vi "Laser Control.vi"(0 "control_laser_source_channel_0_reference":u64 caption="Device In", 1 "control_laser_source_LED_reference":u64 caption="Device In", 2 "control_request":string, 5 "control_laser_source_channel_1_reference":u64 caption="Device In", 7 "control_laser_source_channel_2_reference":u64 caption="Device In", 9 "control_laser_source_channel_3_reference":u64 caption="Device In", 11 "control_laser_source_vibrator_reference":u64 caption="Device In", 12 "control_laser_source":string, 13 "control_laser_source_power":dbl caption="Device In") -> (3 "indicator_light_source_LED_reference":u64 caption="Phidget ID", 4 "indicator_light_source_channel_0_reference":u64 caption="Phidget ID", 6 "indicator_light_source_channel_1_reference":u64 caption="Phidget ID", 8 "indicator_light_source_channel_2_reference":u64 caption="Phidget ID", 10 "indicator_light_source_channel_3_reference":u64 caption="Phidget ID", 14 "indicator_light_source_status":bool caption="Attached?", 15 "indicator_light_source_vibrator_reference":u64 caption="Phidget ID")   [LabVIEW 2020]
uses:
  <vilib>/Utility/file.llb/Read Delimited Spreadsheet (string).vi
  <instrlib>/Phidgets/Phidget Voltage Output/Public/VoltageOutputOpen.vi
  <instrlib>/Phidgets/Phidget Digital Output/Public/DigitalOutputOpen.vi
  <instrlib>/Phidgets/Phidget Voltage Output/Public/VoltageOutputClose.vi
  <instrlib>/Phidgets/Phidget Voltage Output/Phidget Voltage Output.lvlib
  <instrlib>/Phidgets/Phidget Digital Output/Phidget Digital Output.lvlib
panel:
  out "Attached?":bool
  out "error out 12":errorcluster caption="error out"
  out "error out 11":errorcluster caption="error out"
  out "error out 10":errorcluster caption="error out"
  out "error out 9":errorcluster caption="error out"
  out "error out 8":errorcluster caption="error out"
  out "error out 7":errorcluster caption="error out"
  out "error out 6":errorcluster caption="error out"
  out "error out 5":errorcluster caption="error out"
  out "error out 4":errorcluster caption="error out"
  out "error out 3":errorcluster caption="error out"
  out "error out 2":errorcluster caption="error out"
  out "error out":errorcluster
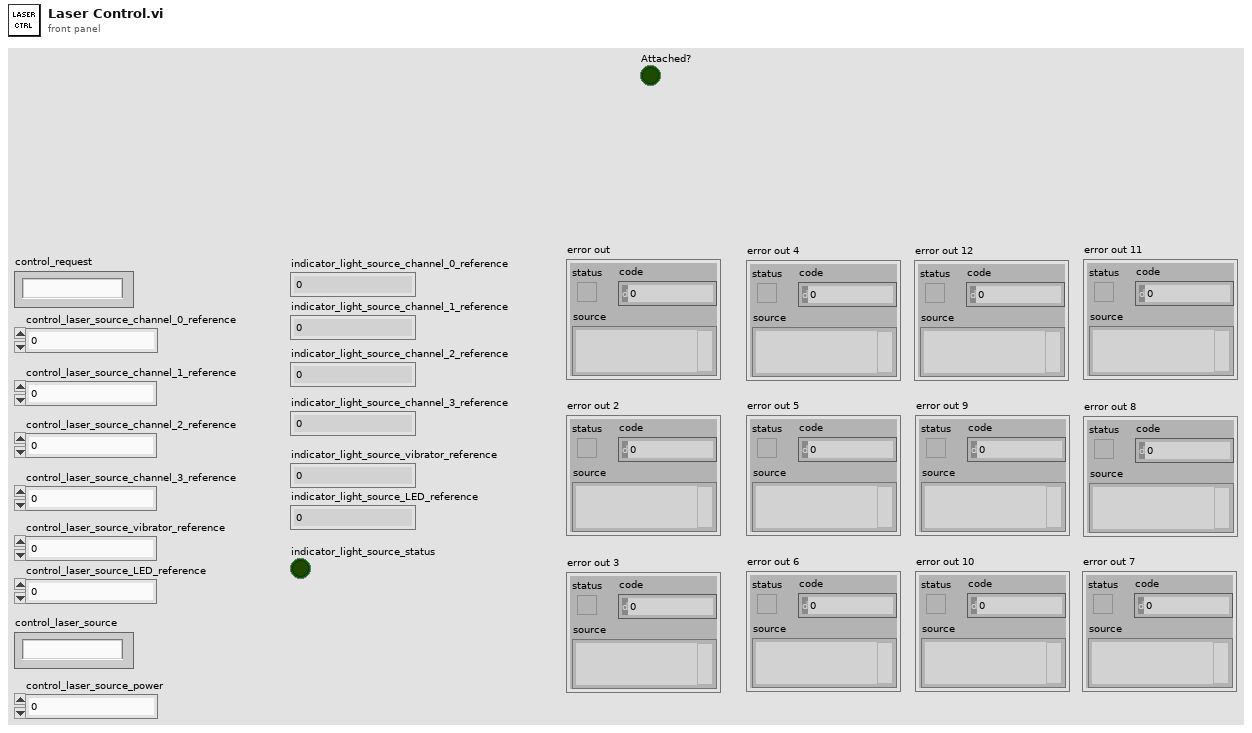
[diagram p1: front panel]
types:
  T1 = cluster{"Serial Number":i32, "Channel":i32, "Port":i32}
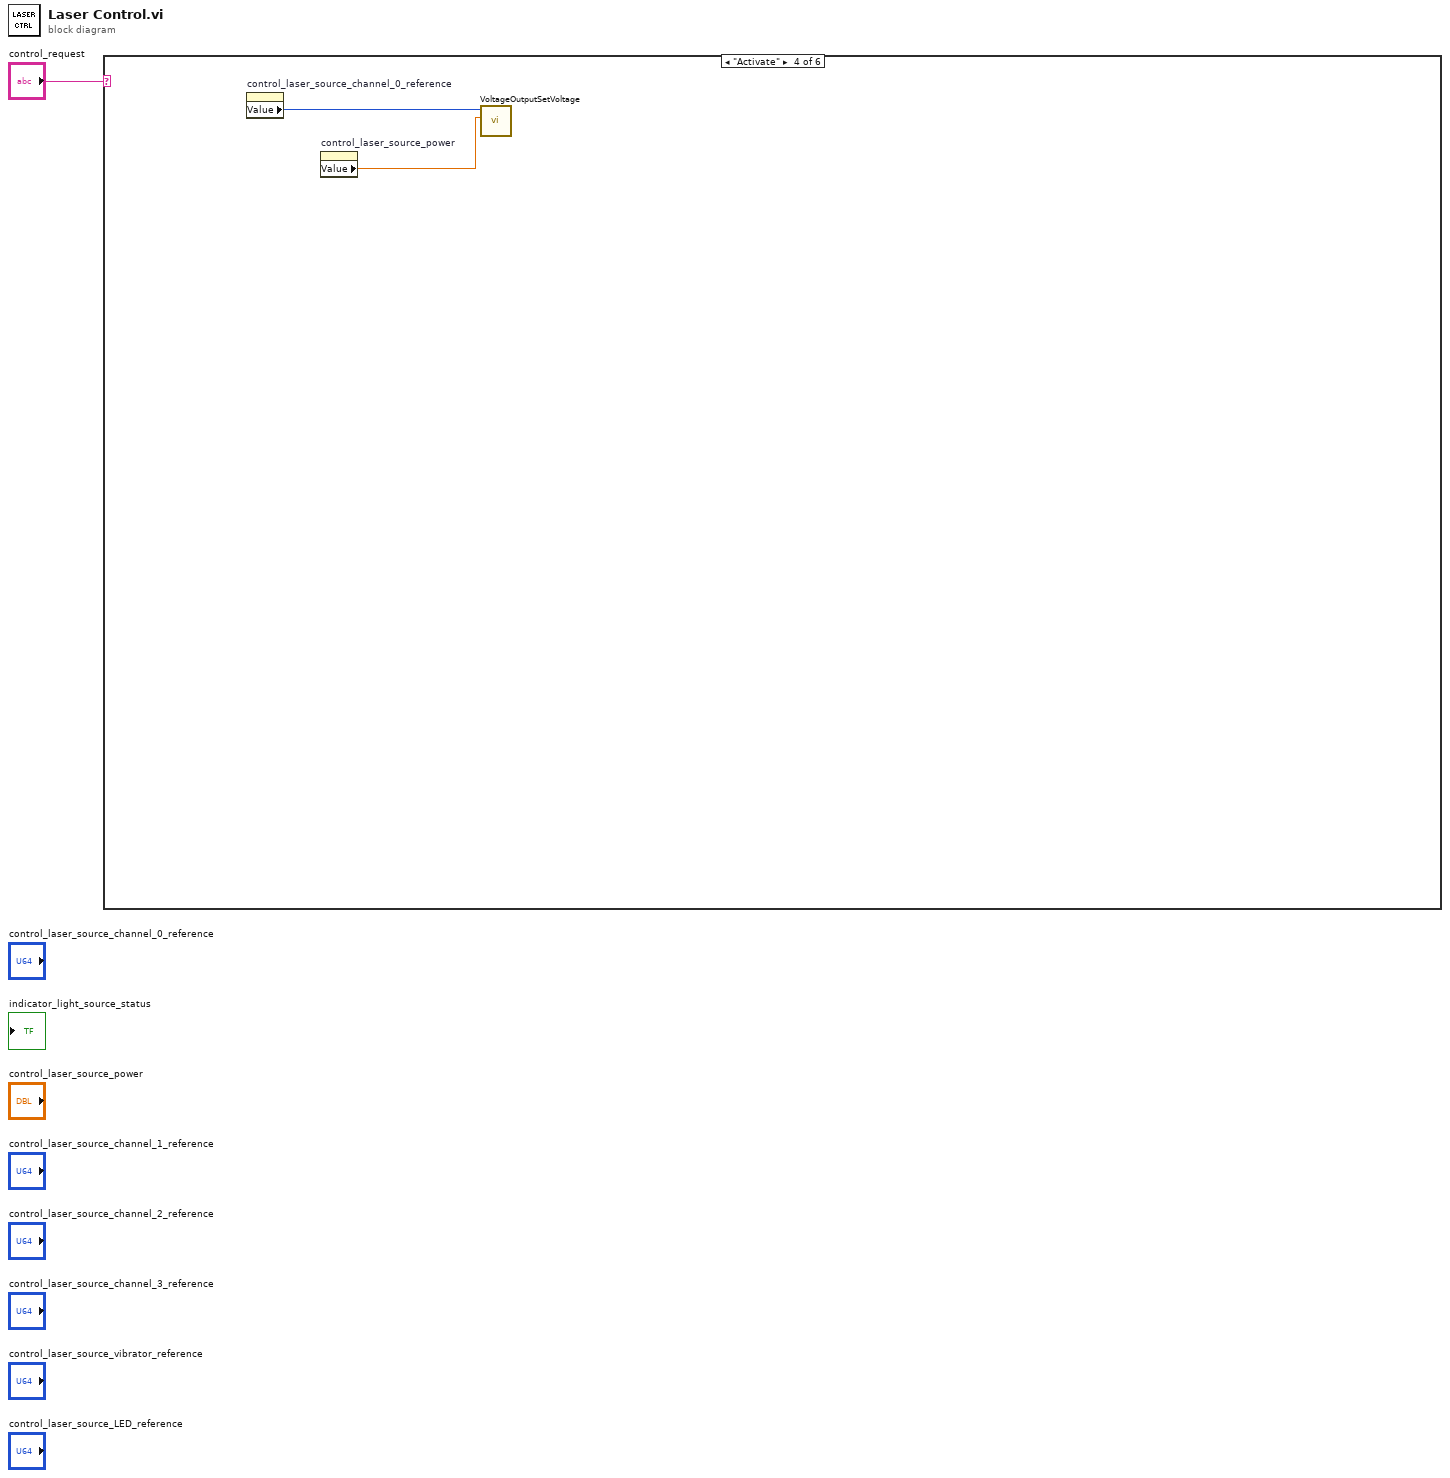
[diagram p0: block diagram]
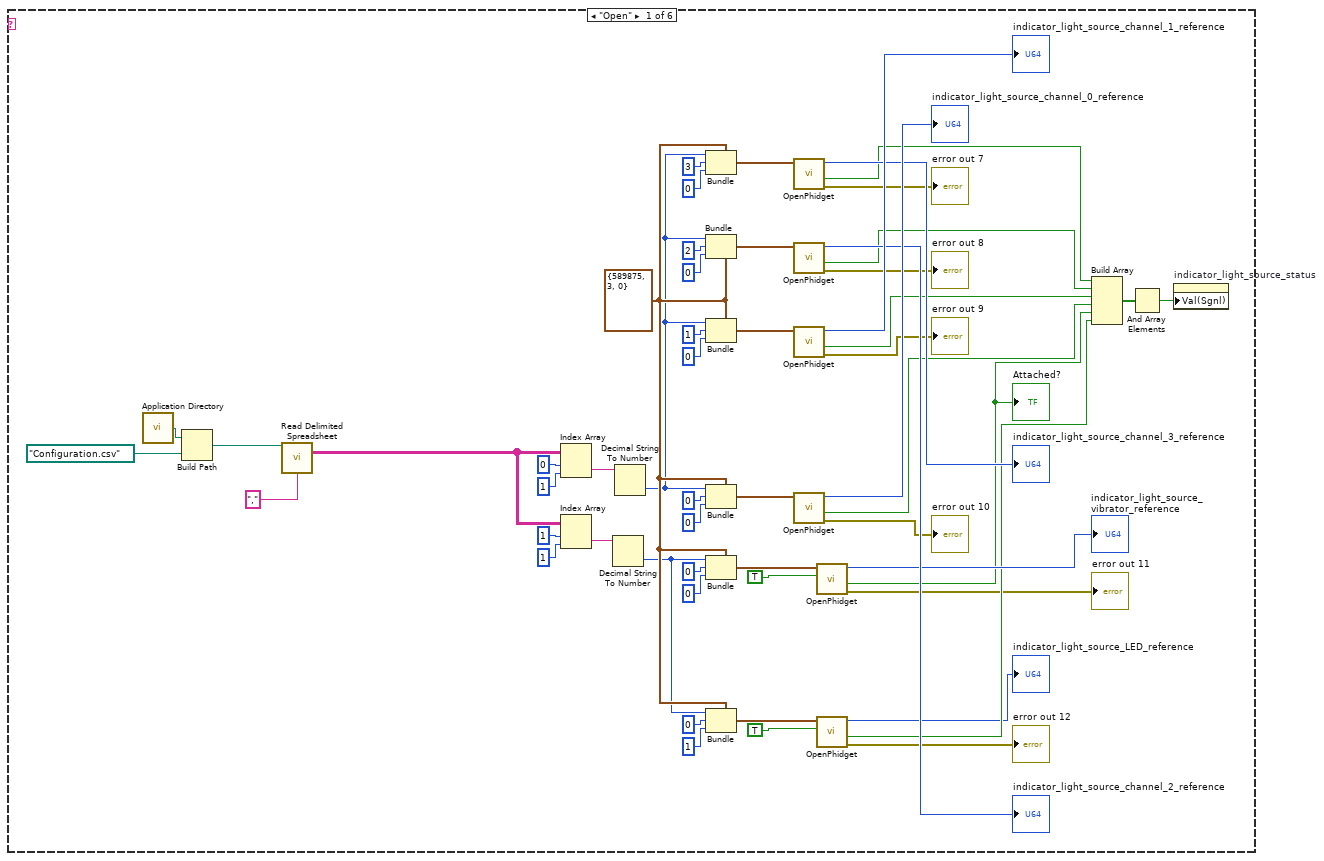
[diagram p2: hidden frame]
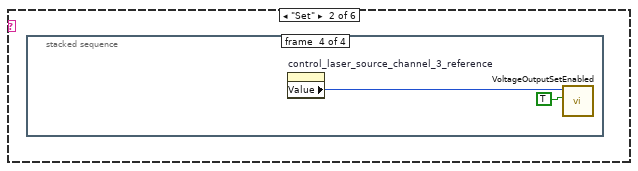
[diagram p3: hidden frame]
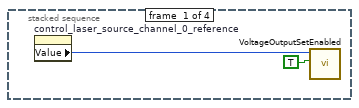
[diagram p4: hidden frame]
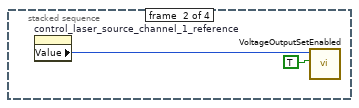
[diagram p5: hidden frame]
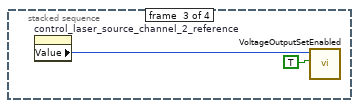
[diagram p6: hidden frame]
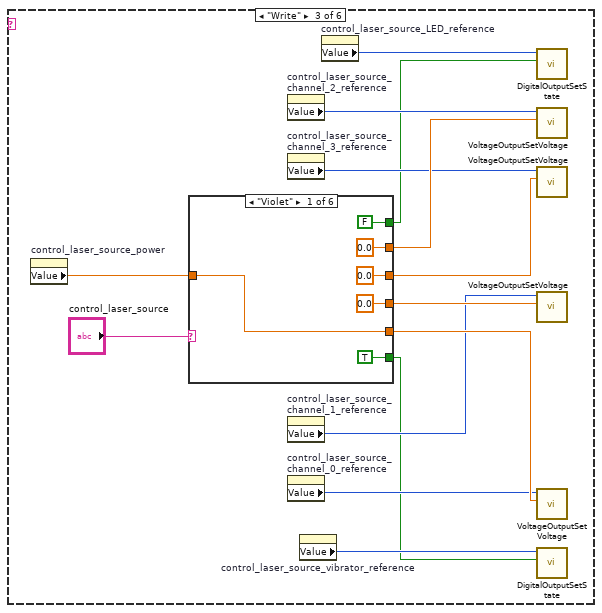
[diagram p7: hidden frame]
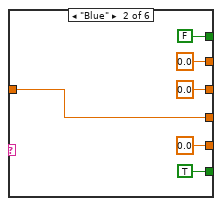
[diagram p8: hidden frame]
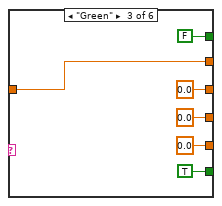
[diagram p9: hidden frame]
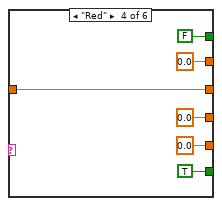
[diagram p10: hidden frame]
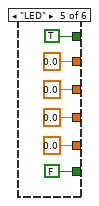
[diagram p11: hidden frame]
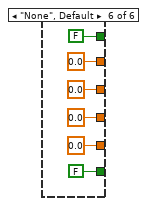
[diagram p12: hidden frame]
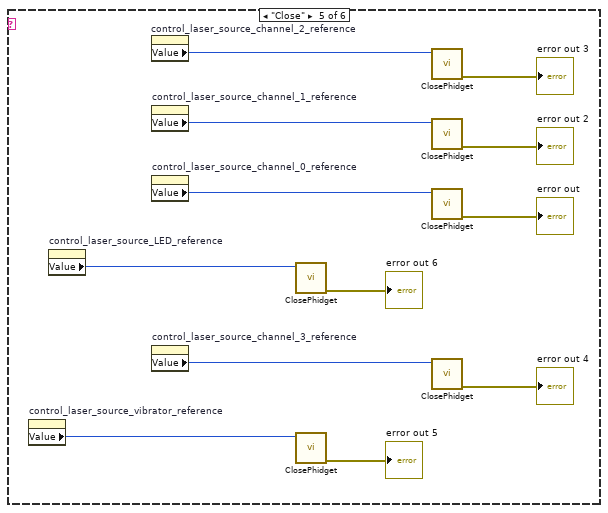
[diagram p13: hidden frame]
diagram:
  n1 = case shown="\"Activate\"" "control_request" {
    frame "Open" {
      w24 = T1 {"Serial Number"=589875, "Channel"=3, "Port"=0} ("Device Info")
      n2 = call <vilib>:"Application Directory.vi"() -> ("Application Directory"=w19:path)
      n3 = Build Path(base path=w19, name or relative path=path "Configuration.csv" ("file path (dialog if empty)")) -> (appended path=w18:path)
      n4 = call-poly <vilib>:"Read Delimited Spreadsheet.vi"("file path (dialog if empty)"=w18, "delimiter (\\t)"="," ("delimiter (\\t)")) -> ("all rows"=w16:string[][])  [unwired: 8 in, 5 out]
      n5 = Index Array(array=w16, index (row)=0, index (col)=1 ("disabled index (col)")) -> (element=w15:string)
      n6 = Index Array(array=w16, index (row)=1, index (col)=1 ("disabled index (col)")) -> (element=w13:string)
      n7 = Decimal String To Number(string=w13) -> (number=w12:i32)  [unwired: 2 in, 1 out]
      n8 = Decimal String To Number(string=w15) -> (number=w14:i32)  [unwired: 2 in, 1 out]
      n9 = Bundle(cluster=w24, "Serial Number"=w14, "Channel"=3, "Port"=0) -> (w39:T1)
      n10 = Bundle(cluster=w24, "Serial Number"=w14, "Channel"=2, "Port"=0) -> (w36:T1)
      n11 = Bundle(cluster=w24, "Serial Number"=w14, "Channel"=1, "Port"=0) -> (w33:T1)
      n12 = Bundle(cluster=w24, "Serial Number"=w14, "Channel"=0, "Port"=0) -> (w30:T1)
      n13 = Bundle(cluster=w24, "Serial Number"=w12, "Channel"=0, "Port"=0) -> (w25:T1)
      n14 = Bundle(cluster=w24, "Serial Number"=w12, "Channel"=0, "Port"=1) -> (w21:T1)
      n15 = call-poly <instrlib>:"OpenPhidget.vi"("Device Info"=w39) -> ("error out"=→"error out 7":errorcluster, "Attached?"=w49:bool, "Phidget ID"=→"indicator_light_source_channel_3_reference":u64)  [unwired: 7 in, 1 out]
      n16 = call-poly <instrlib>:"OpenPhidget.vi"("Device Info"=w36) -> ("error out"=→"error out 8":errorcluster, "Attached?"=w50:bool, "Phidget ID"=→"indicator_light_source_channel_2_reference":u64)  [unwired: 7 in, 1 out]
      n17 = call-poly <instrlib>:"OpenPhidget.vi"("Device Info"=w33) -> ("error out"=→"error out 9":errorcluster, "Attached?"=w5:bool, "Phidget ID"=→"indicator_light_source_channel_1_reference":u64)  [unwired: 7 in, 1 out]
      n18 = call-poly <instrlib>:"OpenPhidget.vi"("Device Info"=w30) -> ("error out"=→"error out 10":errorcluster, "Attached?"=w51:bool, "Phidget ID"=→"indicator_light_source_channel_0_reference":u64)  [unwired: 7 in, 1 out]
      n19 = call-poly <instrlib>:"OpenPhidget.vi"("IsHubPort"=TRUE, "Device Info"=w25) -> ("error out"=→"error out 11":errorcluster, "Attached?"=w4:bool, "Phidget ID"=→"indicator_light_source_vibrator_reference":u64)  [unwired: 6 in, 1 out]
      "Attached?" <- w4
      n20 = call-poly <instrlib>:"OpenPhidget.vi"("IsHubPort"=TRUE, "Device Info"=w21) -> ("error out"=→"error out 12":errorcluster, "Attached?"=w45:bool, "Phidget ID"=→"indicator_light_source_LED_reference":u64)  [unwired: 6 in, 1 out]
      n21 = Build Array(w49, w50, w5, w51, w4, w45) -> (w48:bool[])
      n22 = And Array Elements(Boolean array=w48) -> (logical AND=w47:bool)
      n23 = property on="indicator_light_source_status" class="Bool (strict)"("Val(Sgnl)"=w47) -> ()  [unwired: 2 in, 2 out]
    }
    frame "Set" {
      n24 = stacked-sequence {
        frame #0 {
          n25 = property on="control_laser_source_channel_0_reference" class="DigNum (strict)"() -> ("Value"=w57:u64)  [unwired: 2 in, 2 out]
          n26 = call <instrlib>:"VoltageOutputSetEnabled.vi"("Enabled"=TRUE, "Device In"=w57) -> ()  [unwired: 7 in, 2 out]
        }
        frame #1 {
          n27 = property on="control_laser_source_channel_1_reference" class="DigNum (strict)"() -> ("Value"=w59:u64)  [unwired: 2 in, 2 out]
          n28 = call <instrlib>:"VoltageOutputSetEnabled.vi"("Enabled"=TRUE, "Device In"=w59) -> ()  [unwired: 7 in, 2 out]
        }
        frame #2 {
          n29 = property on="control_laser_source_channel_2_reference" class="DigNum (strict)"() -> ("Value"=w61:u64)  [unwired: 2 in, 2 out]
          n30 = call <instrlib>:"VoltageOutputSetEnabled.vi"("Enabled"=TRUE, "Device In"=w61) -> ()  [unwired: 7 in, 2 out]
        }
        frame #3 {
          n31 = property on="control_laser_source_channel_3_reference" class="DigNum (strict)"() -> ("Value"=w63:u64)  [unwired: 2 in, 2 out]
          n32 = call <instrlib>:"VoltageOutputSetEnabled.vi"("Enabled"=TRUE, "Device In"=w63) -> ()  [unwired: 7 in, 2 out]
        }
      }
    }
    frame "Write" {
      n33 = property on="control_laser_source_power" class="DigNum (strict)"() -> ("Value"=w68:dbl)  [unwired: 2 in, 2 out]
      n34 = case shown="\"Violet\"" "control_laser_source" {
        tunnel: [w80 0.0 ("Voltage") 0.0 ("Voltage") 0.0 ("Voltage") 0.0 ("Voltage") 0.0 ("Voltage")] -> w77
        tunnel: [0.0 ("Voltage") w86 0.0 ("Voltage") 0.0 ("Voltage") 0.0 ("Voltage") 0.0 ("Voltage")] -> w76
        tunnel: [0.0 ("Voltage") 0.0 ("Voltage") w92 0.0 ("Voltage") 0.0 ("Voltage") 0.0 ("Voltage")] -> w75
        tunnel: [0.0 ("Voltage") 0.0 ("Voltage") 0.0 ("Voltage") w98 0.0 ("Voltage") 0.0 ("Voltage")] -> w74
        tunnel: w68 -> [w80 w86 w92 w98 _ _]
        tunnel: [TRUE ("State") TRUE ("State") TRUE ("State") TRUE ("State") FALSE ("State") FALSE ("State")] -> w66
        tunnel: [FALSE ("State") FALSE ("State") FALSE ("State") FALSE ("State") TRUE ("State") FALSE ("State")] -> w64
        frame "Violet" {
        }
        frame "Blue" {
        }
        frame "Green" {
        }
        frame "Red" {
        }
        frame "LED" {
        }
        frame "None", Default {
        }
      }
      n35 = property on="control_laser_source_channel_2_reference" class="DigNum (strict)"() -> ("Value"=w70:u64)  [unwired: 2 in, 2 out]
      n36 = property on="control_laser_source_channel_3_reference" class="DigNum (strict)"() -> ("Value"=w69:u64)  [unwired: 2 in, 2 out]
      n37 = property on="control_laser_source_channel_1_reference" class="DigNum (strict)"() -> ("Value"=w71:u64)  [unwired: 2 in, 2 out]
      n38 = property on="control_laser_source_channel_0_reference" class="DigNum (strict)"() -> ("Value"=w72:u64)  [unwired: 2 in, 2 out]
      n39 = property on="control_laser_source_vibrator_reference" class="DigNum (strict)"() -> ("Value"=w67:u64)  [unwired: 2 in, 2 out]
      n40 = property on="control_laser_source_LED_reference" class="DigNum (strict)"() -> ("Value"=w65:u64)  [unwired: 2 in, 2 out]
      n41 = call <instrlib>:"DigitalOutputSetState.vi"("State"=w64, "Device In"=w65) -> ()  [unwired: 7 in, 2 out]
      n42 = call <instrlib>:"VoltageOutputSetVoltage.vi"("Voltage"=w75, "Device In"=w70) -> ()  [unwired: 7 in, 2 out]
      n43 = call <instrlib>:"VoltageOutputSetVoltage.vi"("Voltage"=w74, "Device In"=w69) -> ()  [unwired: 7 in, 2 out]
      n44 = call <instrlib>:"VoltageOutputSetVoltage.vi"("Voltage"=w76, "Device In"=w71) -> ()  [unwired: 7 in, 2 out]
      n45 = call <instrlib>:"VoltageOutputSetVoltage.vi"("Voltage"=w77, "Device In"=w72) -> ()  [unwired: 7 in, 2 out]
      n46 = call <instrlib>:"DigitalOutputSetState.vi"("State"=w66, "Device In"=w67) -> ()  [unwired: 7 in, 2 out]
    }
    frame "Activate" {
      n47 = property on="control_laser_source_channel_0_reference" class="DigNum (strict)"() -> ("Value"=w115:u64)  [unwired: 2 in, 2 out]
      n48 = property on="control_laser_source_power" class="DigNum (strict)"() -> ("Value"=w114:dbl)  [unwired: 2 in, 2 out]
      n49 = call <instrlib>:"VoltageOutputSetVoltage.vi"("Voltage"=w114, "Device In"=w115) -> ()  [unwired: 7 in, 2 out]
    }
    frame "Close" {
      n50 = property on="control_laser_source_vibrator_reference" class="DigNum (strict)"() -> ("Value"=w119:u64)  [unwired: 2 in, 2 out]
      n51 = property on="control_laser_source_LED_reference" class="DigNum (strict)"() -> ("Value"=w117:u64)  [unwired: 2 in, 2 out]
      n52 = property on="control_laser_source_channel_2_reference" class="DigNum (strict)"() -> ("Value"=w125:u64)  [unwired: 2 in, 2 out]
      n53 = property on="control_laser_source_channel_1_reference" class="DigNum (strict)"() -> ("Value"=w126:u64)  [unwired: 2 in, 2 out]
      n54 = property on="control_laser_source_channel_0_reference" class="DigNum (strict)"() -> ("Value"=w127:u64)  [unwired: 2 in, 2 out]
      n55 = property on="control_laser_source_channel_3_reference" class="DigNum (strict)"() -> ("Value"=w124:u64)  [unwired: 2 in, 2 out]
      n56 = call-poly <instrlib>:"ClosePhidget.vi"("Device In"=w117) -> ("error out"=→"error out 6":errorcluster)  [unwired: 10 in]
      n57 = call-poly <instrlib>:"ClosePhidget.vi"("Device In"=w119) -> ("error out"=→"error out 5":errorcluster)  [unwired: 10 in]
      n58 = call-poly <instrlib>:"ClosePhidget.vi"("Device In"=w125) -> ("error out"=→"error out 3":errorcluster)  [unwired: 10 in]
      n59 = call-poly <instrlib>:"ClosePhidget.vi"("Device In"=w126) -> ("error out"=→"error out 2":errorcluster)  [unwired: 10 in]
      n60 = call-poly <instrlib>:"ClosePhidget.vi"("Device In"=w127) -> ("error out"=→"error out":errorcluster)  [unwired: 10 in]
      n61 = call-poly <instrlib>:"ClosePhidget.vi"("Device In"=w124) -> ("error out"=→"error out 4":errorcluster)  [unwired: 10 in]
    }
    frame "Default", Default {
    }
  }
